vi "Flatten.vi"(8 "error in":errorcluster, 9 "Data":T1) -> (0 "error out":errorcluster, 2 "Buffer":u8[](array[numeric]) format="%.0x")   [LabVIEW 2020, in "GroupData.lvlib"]
uses:
  GroupData.lvlib
  Data.ctl
  <vilib>/IlluminatedG/IG Protoc/LV-Proto/Encode bytes.vi
  <vilib>/IlluminatedG/IG Protoc/LV-Proto/Wire Encode Tag.vi
  <vilib>/IlluminatedG/IG Protoc/LV-Proto/Wire Encode Varint I64.vi
  <vilib>/IlluminatedG/IG Protoc/LV-Proto/Encode LEN.vi
  <vilib>/IlluminatedG/IG Protoc/LV-Proto/Wire Encode Varint I32.vi
  <vilib>/IlluminatedG/IG Protoc/LV-Proto/LV-Proto.lvlib
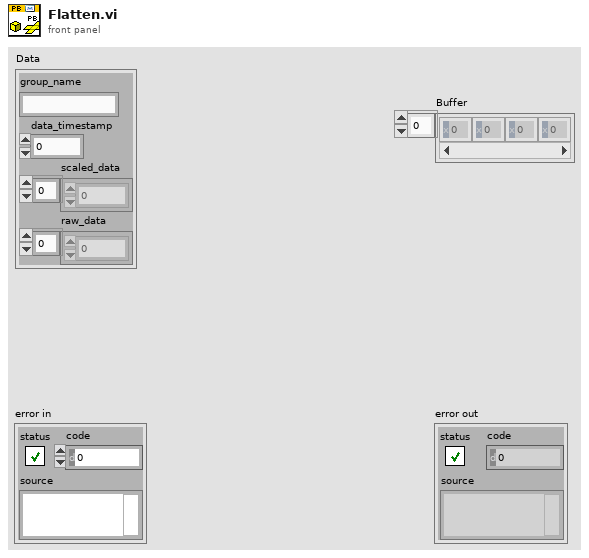
[diagram p1: front panel]
types:
  T1 = typedef "GroupData.lvlib/Data.ctl" = cluster{"group_name":string, "data_timestamp":i64, "scaled_data":dbl[], "raw_data":dbl[]}
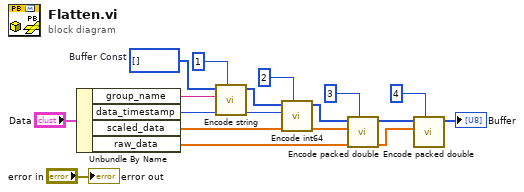
[diagram p0: block diagram]
diagram:
  w13 = u8[] []  # Buffer Const
  n1 = Unbundle By Name("Data") -> ("group_name"=w11:string, "data_timestamp"=w8:i64, "scaled_data"=w5:dbl[], "raw_data"=w2:dbl[])
  n2 = call <vilib>:"Encode string.vi"("Field Number"=1, "string"=w11, "Buffer in"=w13) -> ("Buffer"=w10:u8[])  [unwired: 8 in]
  n3 = call <vilib>:"Encode int64.vi"("Field Number"=2, "int64"=w8, "Buffer in"=w10) -> ("Buffer"=w7:u8[])  [unwired: 8 in]
  n4 = call <vilib>:"Encode packed double.vi"("Field Number"=3, "double"=w5, "Buffer in"=w7) -> ("Buffer"=w4:u8[])  [unwired: 8 in]
  n5 = call <vilib>:"Encode packed double.vi"("Field Number"=4, "double"=w2, "Buffer in"=w4) -> ("Buffer"=→"Buffer":u8[])  [unwired: 8 in]
  "error out" <- "error in"
